vi "replaceDevice.vi"(8 "error in (no error)":errorcluster, 10 "device":refnum<class "device.lvclass">, 11 "DeviceArray in":refnum<class "DeviceArray.lvclass">) -> (0 "error out":errorcluster, 3 "DeviceArray out":refnum<class "DeviceArray.lvclass">)   [LabVIEW 2009, in "Tools.lvlib" / "DatabaseHelpers.lvlib" / "DeviceArray.lvclass"]
uses:
  DeviceArray.lvclass
  device/device.lvclass
  DeviceArray.lvclass/DeviceArray.ctl
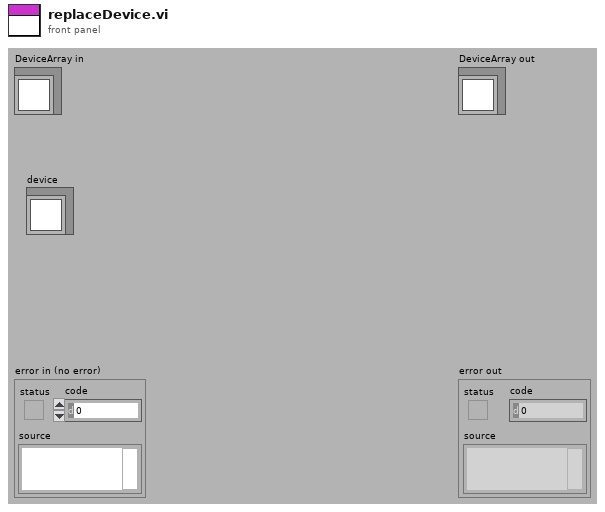
[diagram p1: front panel]
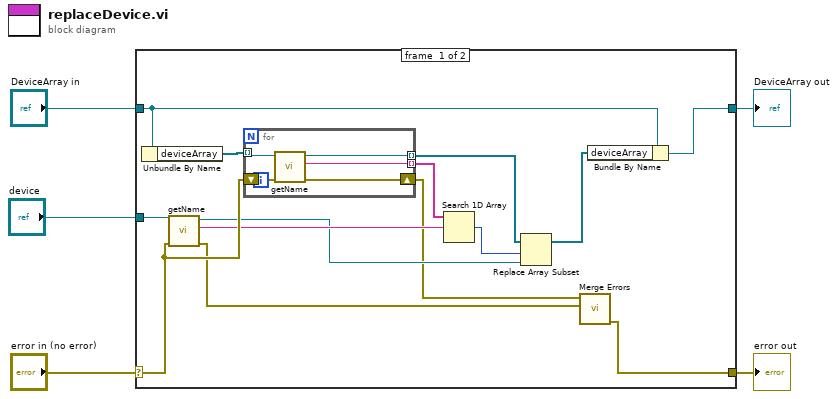
[diagram p0: block diagram]
diagram:
  n1 = case shown="No Error" "error in (no error)" {
    selector: "error in (no error)" -> [w17 w26]
    tunnel: [w6 w26] -> w4
    tunnel: [w10 w25] -> w2
    tunnel: "DeviceArray in" -> [w11 w25]
    tunnel: "device" -> [w19 _]
    frame #0 {
      n2 = Unbundle By Name(w11) -> ("deviceArray"=w18:refnum<class "device.lvclass">[])
      n3 = call "getName.vi"("error in (no error)"=w17, "device.lvclass in"=w19) -> ("error out"=w7:errorcluster, "name"=w15:string, "device.lvclass out"=w12:refnum<class "device.lvclass">)  [unwired: 7 in]
      n4 = for {
        tunnel: w18 -> [w24] mode=indexing
        tunnel: [w22] -> w16 mode=indexing
        tunnel: [w21] -> w14 mode=indexing
        shift-right: [w20] -> w8
        shift-left: w17 -> [w23]
        n5 = call "getName.vi"("error in (no error)"=w23, "device.lvclass in"=w24) -> ("error out"=w20:errorcluster, "name"=w22:string, "device.lvclass out"=w21:refnum<class "device.lvclass">)  [unwired: 7 in]
      }
      n6 = Search 1D Array(1D array=w16, element=w15) -> (index of element=w13:i32)  [unwired: 1 in]
      n7 = Replace Array Subset(array=w14, new element=w12, index=w13) -> (w9:refnum<class "device.lvclass">[])
      n8 = call <vilib>:"Merge Errors.vi"("error in 2 (no error)"=w7, "error in 1 (no error)"=w8) -> ("error out"=w6:errorcluster)  [unwired: 5 in]
      n9 = Bundle By Name(cluster=w11, "deviceArray"=w9) -> (w10:refnum<class "DeviceArray.lvclass">)
    }
    frame #1 {
    }
  }
  "error out" <- w4
  "DeviceArray out" <- w2
